vi "GetInputType.vi"(8 "error in (no error)":errorcluster, 10 "inputIndex":i32, 11 "session id in":i32) -> (0 "error out":errorcluster, 2 "InputTypeIndex":i32, 3 "session id out":i32)   [LabVIEW 2017, in "libonnx_wrapper.lvlib"]
doc: "/**\n * @brief Получить код типа данных входного тензора\n * \n * Возвращает числовой код типа элементов тензора согласно спецификации ONNX.\n * Используйте таблицу констант в начале этого файла для расшифровки.\n * \n * @param sessionId [IN] ID сессии\n * @param inputIndex [IN] Индекс входа (0-based)\n * \n * @return int32: Код типа данных (1=FLOAT32, 2=FLOAT64, 5=INT32, 6=INT64, ...)\n * @return int32: -1 если сессия не найдена или индекс неверен\n * \n * @see GetInputTypeString для получения читаемого имени типа\n */\nint GetInputType(int sessionId, int inputIndex);"
uses:
  libonnx_wrapper.lvlib
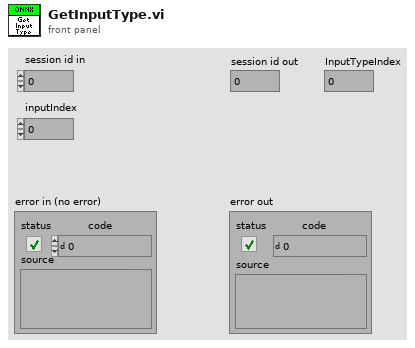
[diagram p1: front panel]
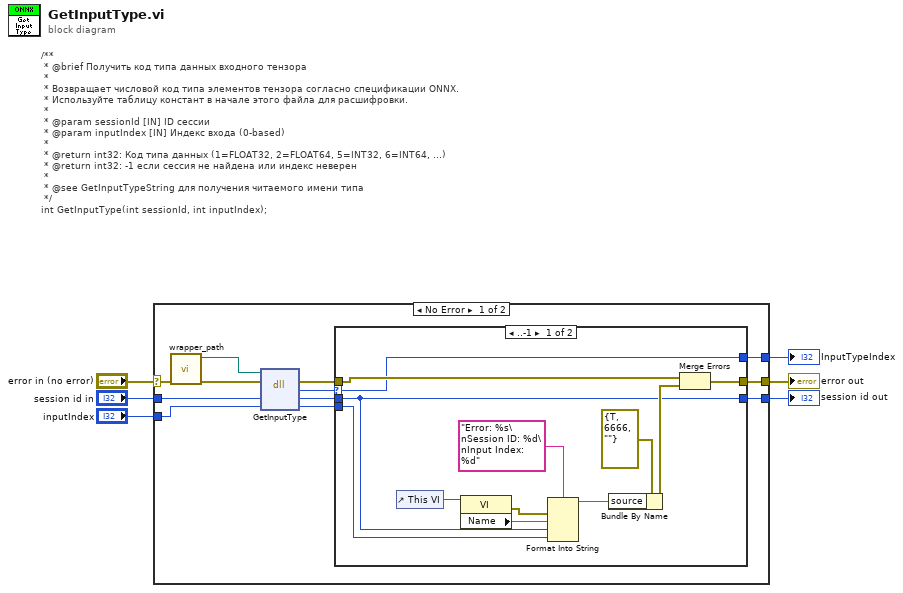
[diagram p0: block diagram]
diagram:
  # "/**\n * @brief Получить код типа данных входного тензора\n * \n * Возвращает числовой код типа элементов тензора согласно спецификации ONNX.\n * Используйте таблицу констант в начале этого файла для расшифровки.\n * \n * @param sessionId [IN] ID сессии\n * @param inputIndex [IN] Индекс входа (0-based)\n * \n * @return int32: Код типа данных (1=FLOAT32, 2=FLOAT64, 5=INT32, 6=INT64, ...)\n * @return int32: -1 если сессия не найдена или индекс неверен\n * \n * @see GetInputTypeString для получения читаемого имени типа\n */\nint GetInputType(int sessionId, int inputIndex);"
  n1 = case shown="No Error" "error in (no error)" {
    selector: "error in (no error)" -> [w7 w35]
    tunnel: "inputIndex" -> [w18 _]
    tunnel: "session id in" -> [w16 w34]
    tunnel: [w12 w35] -> w4
    tunnel: [w11 _] -> w3
    tunnel: [w10 w34] -> w2
    frame No Error {
      n2 = call "wrapper_path.vi"("error in (no error)"=w7) -> ("error out"=w15:errorcluster, "wrapper path"=w17:path)  [unwired: 9 in]
      n3 = dll-call lib="home/ivan/LabVIEWData/ONNX/Test/libonnx_wrapper/unix64/libonnx_wrapper.so" fn="GetInputType"(path in=w17, error in=w15, "sessionId"=w16, "inputIndex"=w18) -> (error out=w14:errorcluster, "InputTypeIndex"=w13:i32, "sessionId"=w9:i32, "inputIndex"=w8:i32)  [unwired: 1 in, 1 out]
      n4 = case shown="..-1" w13 {
        selector: w13 -> [w19 w31]
        tunnel: w14 -> [w21 w33]
        tunnel: [w22 w33] -> w12
        tunnel: w9 -> [w23 w32]
        tunnel: [w23 w32] -> w10
        tunnel: w8 -> [w20 _]
        tunnel: [w19 w31] -> w11
        frame ..-1 {
          n5 = control-ref of="This VI"() -> (w27:refnum<vi>)
          n6 = property class="VI"(reference=w27) -> (error out=w24:errorcluster, "Name"=w26:string)  [unwired: 1 in, 1 out]
          n7 = Format Into String(format string="Error: %s\nSession ID: %d\nInput Index: %d", error in=w24, w26, w23, w20) -> (resulting string=w28:string)  [unwired: 1 in, 1 out]
          n8 = Bundle By Name(cluster=errorcluster {"status"=TRUE, "code"=6666, "source"=""} ("error out"), "source"=w28) -> (w29:errorcluster)
          n9 = Merge Errors(w21, w29) -> (w22:errorcluster)
        }
        frame 0.. {
        }
      }
    }
    frame Error {
    }
  }
  "error out" <- w4
  "session id out" <- w2
  "InputTypeIndex" <- w3
